vi "fgv.vi"(8 "error in (no error)":errorcluster, 10 "R/W (Write = True)":bool=TRUE, 11 "Flag":bool) -> (0 "error out":errorcluster, 3 "Flag out":bool)   [LabVIEW 2020]
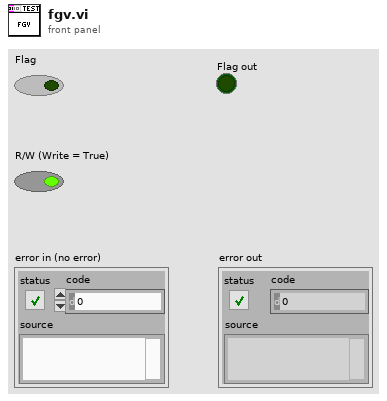
[diagram p1: front panel]
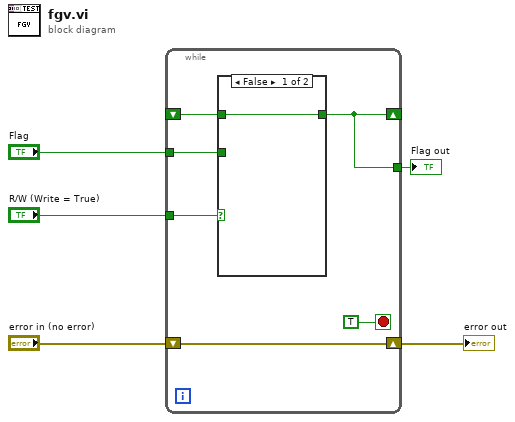
[diagram p0: block diagram]
diagram:
  n1 = while {
    shift-right: [w11] -> w4
    shift-left: "error in (no error)" -> [w11]
    tunnel: "R/W (Write = True)" -> [w9]
    tunnel: "Flag" -> [w8]
    shift-right: [w6] -> _
    shift-left: _ -> [w7]
    tunnel: [w6] -> w1
    stop <- TRUE stop-if-true
    n2 = case shown="False" w9 {
      tunnel: w8 -> [_ w13]
      tunnel: [w12 w13] -> w6
      tunnel: w7 -> [w12 _]
      frame False {
      }
      frame True {
      }
    }
  }
  "error out" <- w4
  "Flag out" <- w1
